vi "Teleop.vi"(10 "Match Info":T1={"Autonomous Elapsed Seconds"=0.0, "TeleOp Elapsed Seconds"=0.0, "Disabled Elapsed Seconds"=0.0, "Visited Autonomous"=FALSE, "Visited TeleOp"=FALSE, "Visited Disabled"=FALSE, "Autonomous Settings"={"Autonomous Style"=enum."Independent", "VI Refnum"=refnum}}, 11 "Call Context":T2) -> ()   [LabVIEW 2017]
doc: "This VI is called for each TeleOp packet received from the DS where the robot is not disabled. It is often used to read from the joysticks and update I/O or to update setpoints for timed control loops. It should complete and return within 20 milliseconds or it may miss DS packets."
uses:
  <vilib>/Rock Robotics/WPI/DriverStation/WPI_DriverStationDerivedRobotMode.ctl
  <vilib>/Rock Robotics/WPI/DriverStation/WPI_DriverStationMatch Info.ctl
  <vilib>/Rock Robotics/WPI/Solenoid/WPI_SolenoidValue.ctl
  <vilib>/Rock Robotics/Network Tables/NT Write Numeric Array.vi
  <vilib>/Rock Robotics/Network Tables/NT Write Boolean Array.vi
  Robot Global Data.vi
  <vilib>/Rock Robotics/Network Tables/NT Read Boolean.vi
  <vilib>/Rock Robotics/Network Tables/NT Read String.vi
  <vilib>/Rock Robotics/WPI/Utilities/WPI_GetSetVariantRefNum.vi
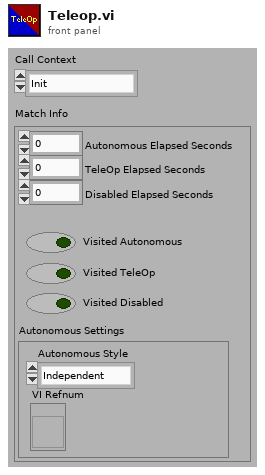
[diagram p1: front panel]
types:
  T1 = typedef "WPI_DriverStationMatch Info.ctl" = cluster{"Autonomous Elapsed Seconds":dbl, "TeleOp Elapsed Seconds":dbl, "Disabled Elapsed Seconds":dbl, "Visited Autonomous":bool, "Visited TeleOp":bool, "Visited Disabled":bool, "Autonomous Settings":cluster{"Autonomous Style":enum16{"Iterative", "Independent"}, "VI Refnum":refnum<vi>}}
  T2 = typedef "WPI_DriverStationDerivedRobotMode.ctl" = enum16{"Init", "Execute", "Stop"}
  T3 = enum16{"1 Xbox Controller", "2 Xbox Controllers"}
  T4 = typedef "TeleopCommands.ctl" = cluster{"Drive Axes":dbl[], "Shooter Forwards":bool, "Shooter Reverse":bool, "Intake Forwards":bool, "Intake Reverse":bool, "Lift Forwards":bool, "Lift Reverse":bool, "Agitator Forwards":bool, "Agitator Reverse":bool, "Left Gear Angle":bool, "Mid Gear Angle":bool, "Right Gear Angle":bool, "Shooter Distance":bool, "Vision Align":bool, "Place Gear":bool, "Command Stop":bool, "Reset Gyro":bool, "Jog Mode?":bool, "Lift Override":bool, "Lift Power":dbl}
  T5 = typedef "WPI_JoystickDevRef.ctl" = cluster{"Device":T6}
  T6 = typedef "WPI_JoystickDeviceEnum.ctl" = enum16{"USB 0", "USB 1", "USB 2", "USB 3", "USB 4", "USB 5"}
  T7 = cluster{"Yaw":dbl, "Roll":dbl, "Pitch":dbl, "Heading":dbl, "Fused Heading":dbl}
  T8 = typedef "WPI_MotorControlDeviceRef.ctl" = cluster{"DeviceStatus":errorcluster, "Type":T9, "PWM":cluster{"PWM Channel":T10, "DeadBand":T11}, "CAN":cluster{"Device Number":u8, "SetOutput VI Ref":variant, "GetOutput VI Ref":variant, "Enable VI Ref":variant, "Disable VI Ref":variant, "Data":variant}, "Invert":bool, "DIO PWM":cluster{"PWM \"Enable\" Channel":T10, "DIOChannel":T12, "PWM Rate":dbl}}
  T9 = typedef "WPI_MotorControlType.ctl" = enum16{"PWM", "CAN", "DIO PWM"}
  T10 = typedef "FPGA_DIOPWMChannel.ctl" = enum8{"PWM 0", "PWM 1", "PWM 2", "PWM 3", "PWM 4", "PWM 5", "PWM 6", "PWM 7", "PWM 8", "PWM 9", "PWM MXP 0", "PWM MXP 1", "PWM MXP 2", "PWM MXP 3", "PWM MXP 4", "PWM MXP 5", "PWM MXP 6", "PWM MXP 7", "PWM MXP 8", "PWM MXP 9", "Invalid"}
  T11 = typedef "WPI_PWMDeadband.ctl" = cluster{"Name":string, "maxPositivePwm":i32, "minPositivePwm":i32, "centerPwm":i32, "maxNegativePwm":i32, "minNegativePwm":i32, "angularRange":u16}
  T12 = typedef "FPGA_DIOChannel.ctl" = enum8{"DIO 0", "DIO 1", "DIO 2", "DIO 3", "DIO 4", "DIO 5", "DIO 6", "DIO 7", "DIO 8", "DIO 9", "DIO MXP 0", "DIO MXP 1", "DIO MXP 2", "DIO MXP 3", "DIO MXP 4", "DIO MXP 5", "DIO MXP 6", "DIO MXP 7", "DIO MXP 8", "DIO MXP 9", "DIO MXP 10", "DIO MXP 11", "DIO MXP 12", "DIO MXP 13", "DIO MXP 14", "DIO MXP 15", "SPI Port CS1", "SPI Port CS2", "SPI Port CS3", "SPI Port MISO", "SPI Port MOSI", "Invalid"}
  T13 = typedef "WPI_SolenoidValue.ctl" = enum16{"Off", "On", "Forward", "Reverse"}
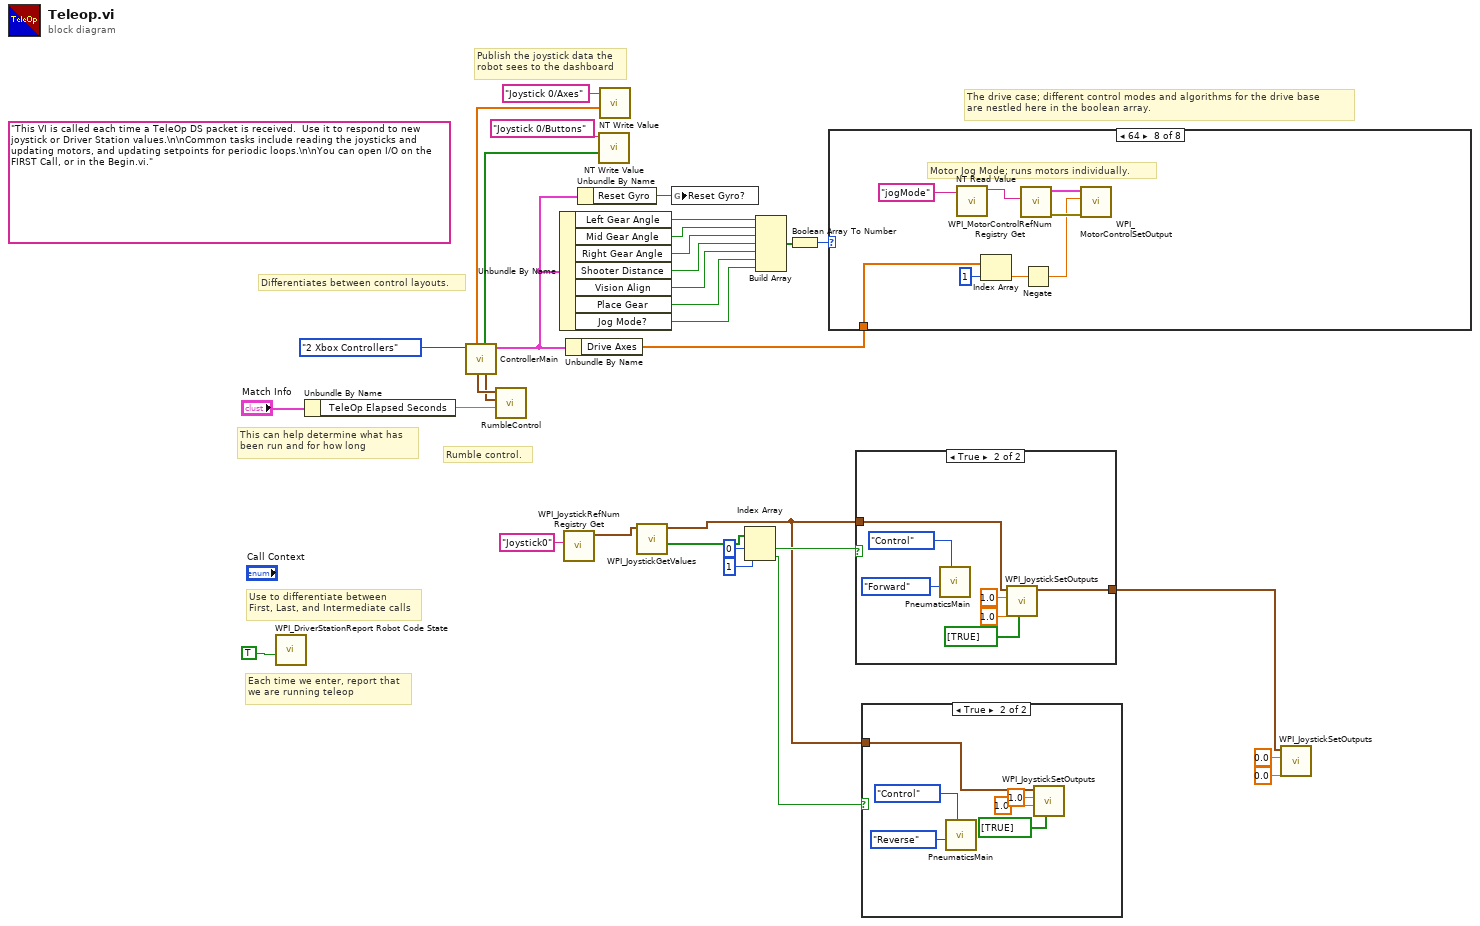
[diagram p0: block diagram]
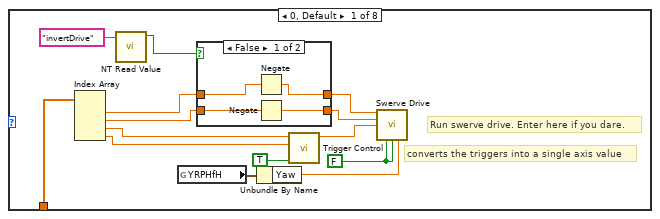
[diagram p4: hidden frame]
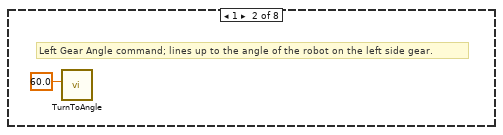
[diagram p6: hidden frame]
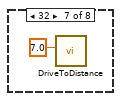
[diagram p11: hidden frame]
diagram:
  (unwired) "This VI is called each time a TeleOp DS packet is received.  Use it to respond to new joystick or Driver Station values.\n\nCommon tasks include reading the joysticks and updating motors, and updating setpoints for periodic loops.\n\nYou can open I/O on the FIRST Call, or in the Begin.vi."
  # "The drive case; different control modes and algorithms for the drive base \nare nestled here in the boolean array."
  # "Rumble control."
  # "Differentiates between control layouts."
  # "Publish the joystick data the\nrobot sees to the dashboard"
  # "Each time we enter, report that\nwe are running teleop"
  # "Use to differentiate between\nFirst, Last, and Intermediate calls"
  # "This can help determine what has\nbeen run and for how long"
  n1 = call <vilib>:"WPI_DriverStationReport Robot Code State.vi"("TeleOp"=TRUE ("Autonomous")) -> ()  [unwired: 10 in, 1 out]
  n2 = Unbundle By Name("Match Info") -> ("TeleOp Elapsed Seconds"=w22:dbl)
  n3 = call "ControllerMain.vi"("Control Mode"=T3."2 Xbox Controllers") -> ("Robot Inputs"=w20:T4, "Joystick1DevRef"=w23:T5, "Stick0 Buttons"=w26:bool[], "Joystick0DevRef"=w24:T5, "Stick0 Axes"=w27:dbl[])  [unwired: 5 in, 1 out]
  n4 = call "RumbleControl.vi"("Teleop Time"=w22, "JoystickDevRef1"=w23, "JoystickDevRef0"=w24) -> ()  [unwired: 8 in, 1 out]
  n5 = Unbundle By Name(w20) -> ("Left Gear Angle"=w19:bool, "Mid Gear Angle"=w18:bool, "Right Gear Angle"=w17:bool, "Shooter Distance"=w16:bool, "Vision Align"=w15:bool, "Place Gear"=w14:bool, "Jog Mode?"=w12:bool)
  n6 = call <vilib>:"WPI_JoystickRefNum Registry Get.vi"("refnum name"="Joystick0") -> ("JoystickDevRef"=w10:T5)  [unwired: 9 in, 1 out]
  n7 = Unbundle By Name(w20) -> ("Drive Axes"=w29:dbl[])
  n8 = Unbundle By Name(w20) -> ("Reset Gyro"=w13:bool)
  n9 = call-poly <vilib>:"NT Write Value.vi"("Boolean Array"=w26, "Name"="Joystick 0/Buttons") -> ()  [unwired: 9 in, 1 out]
  n10 = call-poly <vilib>:"NT Write Value.vi"("Numeric Array"=w27, "Name"="Joystick 0/Axes") -> ()  [unwired: 9 in, 1 out]
  n11 = call <vilib>:"WPI_JoystickGetValues.vi"("JoystickDevRef"=w10) -> ("Buttons"=w9:bool[], "JoystickDevRef"=w3:T5)  [unwired: 6 in, 3 out]
  n12 = global write "Robot Global Data.vi" "Reset Gyro?"(w13) -> ()
  n13 = Index Array(array=w9, index #1=0 ("index"), index #2=1 ("index")) -> (element #1=w7:bool, element #2=w5:bool)
  n14 = Build Array(w19, w18, w17, w16, w15, w14, w12) -> (w25:bool[])
  n15 = Boolean Array To Number(Boolean array=w25) -> (number=w21:u32)
  n16 = case shown="64" w21 {
    tunnel: w29 -> [w47 _ _ _ _ _ _ w63]
    frame 0, Default {
      w40 = FALSE ("Robot Centric?")
      # "converts the triggers into a single axis value"
      # "Run swerve drive. Enter here if you dare."
      n17 = Index Array(array=w47) -> (element #1=w39:dbl, element #2=w38:dbl, element #3=w46:dbl, element #4=w45:dbl)  [unwired: 4 in]
      n18 = call-poly <vilib>:"NT Read Value.vi"("Name"="invertDrive") -> ("Boolean"=w34:bool)  [unwired: 9 in, 1 out]
      n19 = global read "Robot Global Data.vi" "YRPHfH"() -> (w42:T7)
      n20 = case shown="False" w34 {
        tunnel: w39 -> [w51 w53]
        tunnel: w38 -> [w50 w52]
        tunnel: [w49 w53] -> w37
        tunnel: [w48 w52] -> w36
        frame False {
          n21 = Negate(x=w51) -> (-x=w49:dbl)
          n22 = Negate(x=w50) -> (-x=w48:dbl)
        }
        frame True {
        }
      }
      n23 = Unbundle By Name(w42) -> ("Yaw"=w41:dbl)
      n24 = call "Trigger Control.vi"("Invert?"=TRUE, "Axis 2 In"=w45, "Axis 1 In"=w46) -> ("Axis Out"=w43:dbl)  [unwired: 8 in]
      n25 = call "Swerve Drive.vi"("X"=w37, "Y"=w36, "Z"=w43, "Robot Centric?"=w40, "Autonomous?"=w40, "Yaw"=w41) -> ()  [unwired: 5 in, 5 out]
    }
    frame 1 {
      # "Left Gear Angle command; lines up to the angle of the robot on the left side gear."
      n26 = call "TurnToAngle.vi"("Target Angle"=60.0) -> ()  [unwired: 10 in, 1 out]
    }
    frame 2 {
      # "Middle Gear command: Lines up to the gear on the middle"
    }
    frame 4 {
      # "Right Gear Angle: Lines up to the right side gear peg."
    }
    frame 8 {
      # "Shooter Distance: Drives until aligned to the"
    }
    frame 16 {
    }
    frame 32 {
      n27 = call "DriveToDistance.vi"("Setpoint"=7.0) -> ()  [unwired: 10 in, 1 out]
    }
    frame 64 {
      # "Motor Jog Mode; runs motors individually."
      n28 = call-poly <vilib>:"NT Read Value.vi"("Name"="jogMode") -> ("String"=w60:string)  [unwired: 9 in, 1 out]
      n29 = Index Array(array=w63, index=1) -> (element=w61:dbl)
      n30 = call <vilib>:"WPI_MotorControlRefNum Registry Get.vi"("refnum name"=w60) -> ("error out"=w59:errorcluster, "MotorControlDevRef"=w58:T8)  [unwired: 9 in]
      n31 = Negate(x=w61) -> (-x=w57:dbl)
      n32 = call <vilib>:"WPI_MotorControlSetOutput.vi"("error in (no error)"=w59, "Output"=w57, "MotorControlDevRef"=w58) -> ()  [unwired: 6 in, 3 out]
    }
  }
  n33 = case shown="True" w7 {
    tunnel: w3 -> [w64 w69]
    tunnel: [w64 w66] -> w4
    frame False {
    }
    frame True {
      n34 = call "PneumaticsMain.vi"("Mode"=enum16{"Open", "Control"}."Control", "Value"=WPI_SolenoidValue."Forward") -> ()  [unwired: 9 in, 1 out]
      n35 = call <vilib>:"WPI_JoystickSetOutputs.vi"("Outputs"=bool[] [TRUE], "Right Rumble"=sgl 1.0, "Left Rumble"=sgl 1.0, "JoystickDevRef"=w69) -> ("JoystickDevRef"=w66:T5)  [unwired: 6 in, 1 out]
    }
  }
  n36 = case shown="True" w5 {
    tunnel: w3 -> [_ w75]
    frame False {
    }
    frame True {
      n37 = call "PneumaticsMain.vi"("Mode"=enum16{"Open", "Control"}."Control", "Value"=WPI_SolenoidValue."Reverse") -> ()  [unwired: 9 in, 1 out]
      n38 = call <vilib>:"WPI_JoystickSetOutputs.vi"("Outputs"=bool[] [TRUE], "Right Rumble"=sgl 1.0, "Left Rumble"=sgl 1.0, "JoystickDevRef"=w75) -> ()  [unwired: 6 in, 2 out]
    }
  }
  n39 = call <vilib>:"WPI_JoystickSetOutputs.vi"("Right Rumble"=sgl 0.0, "Left Rumble"=sgl 0.0, "JoystickDevRef"=w4) -> ()  [unwired: 7 in, 2 out]
